vi "GetDecimation.vi"(8 "error in (no error)":errorcluster, 11 "reference in":refnum<class "Fcurve.lvclass">) -> (0 "error out":errorcluster, 2 "Decimation":T1={"App"={"Dec"=1, "apply"=FALSE}, "Con"={"Dec"=1, "apply"=FALSE}, "Ret"={"Dec"=1, "apply"=FALSE}}, 3 "reference out":refnum<class "Fcurve.lvclass">)   [LabVIEW 2019, in "Fcurve.lvclass"]
uses:
  Fcurve.lvclass
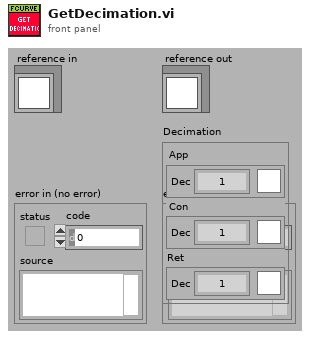
[diagram p1: front panel]
types:
  T1 = cluster{"App":cluster{"Dec":i32, "apply":bool}, "Con":cluster{"Dec":i32, "apply":bool}, "Ret":cluster{"Dec":i32, "apply":bool}}
  T2 = typedef "Fcurve.lvclass/ObjectAttributesRef.ctl" = refnum<data-value>
  T3 = typedef "Fcurve.lvclass/ObjectAttributes.ctl" = cluster{"MyAttribute":dbl, "Fcurve Metadata":T4, "Contact Spread of dev":dbl, "Tau Delay (ms)":dbl, "Points of contact":dbl, "Def_wfm":cluster{"Max":dbl, "Min":dbl}, "Zpos_wfm":cluster{"Max":dbl, "Min":dbl}, "Contact stat?":bool, "Real AI dt (s)":dbl, "Decimation":cluster{"App":cluster{"Dec":i32, "apply":bool}, "Con":cluster{"Dec":i32, "apply":bool}, "Ret":cluster{"Dec":i32, "apply":bool}}, "Segment def[0]":dbl, "Segment Zpos[0]":dbl, "Raw Datum":waveform(dbl)[], "Group metadata":T5, "M_data obj":refnum<class "metadata.lvclass">, "Channel name(s)":string[], "Segment fcurve data":cluster{"X":dbl[], "Y":dbl[]}[], "Segment duration":cluster{"Start":i32, "Duration":i32}[], "Segment info":T6[], "Segment durations (S)":dbl[], "Segments Maxmin":T8[]}
  T4 = typedef "Fcurve.lvclass/Metadata.ctl" = cluster{"dt (us)":dbl, "Dec Factor":dbl, "Z piezo Sensitivity (nm/V)":dbl, "K (N/m)":dbl, "Sp (V)":dbl, "Contact (ms)":dbl, "Zpos contact":dbl, "Vel_app (nm/s)":dbl, "Vel_ret (nm/s)":dbl, "deltaV (nm)":dbl, "Def_V0 (v)":dbl, "Piezo gain":dbl, "invOLS (nm/V)":dbl}
  T5 = typedef "TDMS_DataHandler.lvclass/Fcurve Meta data.ctl" = cluster{"property names":string[], "property values":variant[]}
  T6 = typedef "Fcurve.lvclass/Fcurve segments --cluster.ctl" = cluster{"type":T7, "nb points":i32, "dec factor":u32, "sampling rate (S/s)":u32}
  T7 = typedef "metadata.lvclass/Segment type--combobox.ctl" = string
  T8 = typedef "Fcurve.lvclass/Segment MaxMin --cluster.ctl" = cluster{"Def":cluster{"max value":dbl, "min value":dbl}, "Zpos":cluster{"max value":dbl, "min value":dbl}}
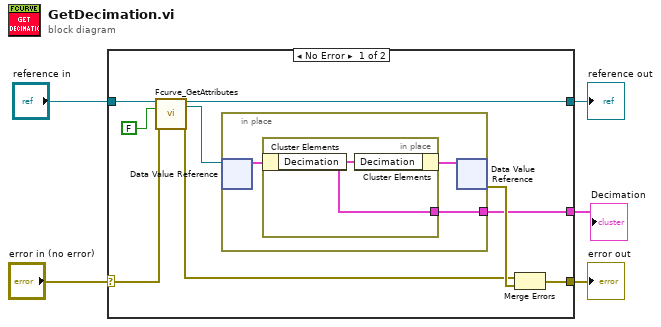
[diagram p0: block diagram]
diagram:
  n1 = case shown="No Error" "error in (no error)" {
    selector: "error in (no error)" -> [w14 w20]
    tunnel: [w8 w20] -> w4
    tunnel: [w13 w19] -> w2
    tunnel: "reference in" -> [w12 w19]
    tunnel: [w6 _] -> w1
    frame No Error {
      n2 = call "Fcurve_GetAttributes.vi"("reference in"=w12, "return data? (T)"=FALSE, "error in (no error)"=w14) -> ("reference out"=w13:refnum<class "Fcurve.lvclass">, "attributes ref"=w7:T2, "error out"=w9:errorcluster)  [unwired: 13 in, 1 out]
      n3 = in-place {
        in-place-border: [w15] -> w6
        n4 = in-place-dvr #1(w7) -> (w16:T3)  [unwired: 1 out]
        n5 = in-place {
          in-place-border: [w18] -> w15
          n6 = in-place-cluster #2(w16) -> ("Decimation"=w18:T1)
          n7 = in-place-cluster #2("Decimation"=w18) -> (w17:T3)
        }
        n8 = in-place-dvr #1(w17) -> (w10:errorcluster)  [unwired: 1 out]
      }
      n9 = Merge Errors(w9, w10) -> (w8:errorcluster)
    }
    frame Error {
    }
  }
  "error out" <- w4
  "reference out" <- w2
  "Decimation" <- w1
